vi "FFT_test.vi"() -> ()   [LabVIEW 2009]
uses:
  <vilib>/imath/engines/lvmath2/RunTimeEngine/ErrorHandling/NIMS_Finalize Error.vi
  <vilib>/imath/engines/lvmath2/RunTimeEngine/Parser/MC_Version.vi
  <vilib>/imath/engines/lvmath2/RunTimeEngine/NodeEndStatement/NIMS_NodeEndStatement_Output.vi
  <instcachedir>/0/NIMS_NodeEndStatement_Output_53EC0D466D134D7ABD903AC30B43404B.lvgen/NIMS_NodeEndStatement_Output_53EC0D466D134D7ABD903AC30B43404B_001.vi
  <vilib>/imath/engines/lvmath2/RunTimeEngine/RangeToken/NIMS_Range.vi
  <instcachedir>/0/NIMS_Range_08574DECC23E450FAF0AC0BC39E6BEA7.lvgen/NIMS_Range_08574DECC23E450FAF0AC0BC39E6BEA7_000.vi
  <vilib>/imath/engines/lvmath/Functions/Error Handling/MergeErrorsWrapper.vi
  <vilib>/imathl/engines/lvmath/Functions/Error Handling/Create Error.vi
  <vilib>/imath/engines/lvmath/Functions/Error Handling/MC_Error Cluster From Error Code.vi
  <vilib>/imath/engines/lvmath2/RunTimeEngine/BuiltInFunctions/randnormal/NIMS_randnormal(1,I32).vi
  <vilib>/imath/engines/lvmath2/RunTimeEngine/ArithmeticOperatorToken/NIMS_ArithmeticOperator_power(S).vi
  <instcachedir>/0/NIMS_ArithmeticOperator_power(S)_4AA2794EBDEE41D3AEDF40937D3906E7.lvgen/NIMS_ArithmeticOperator_power(S)_4AA2794EBDEE41D3AEDF40937D3906E7_001.vi
  <vilib>/imath/engines/lvmath2/RunTimeEngine/BuiltInFunctions/fft/NIMS_fft(GV).vi
  <instcachedir>/0/NIMS_fft(GV)_4C6467FC22F84E4BA42517A07EF978B0.lvgen/NIMS_fft(GV)_4C6467FC22F84E4BA42517A07EF978B0_001.vi
  <vilib>/imath/engines/lvmath2/RunTimeEngine/BuiltInFunctions/abs/NIMS_abs(signed).vi
  <instcachedir>/0/NIMS_abs(signed)_C4FCB8E6058B49B797C7C8D53CA5F6EC.lvgen/NIMS_abs(signed)_C4FCB8E6058B49B797C7C8D53CA5F6EC_000.vi
panel:
  out "FFT of 1023 Pt Sequence":cluster{dbl[], dbl[]}(graph)
  out "Time Domain Sequence":cluster{dbl[], dbl[]}(graph)
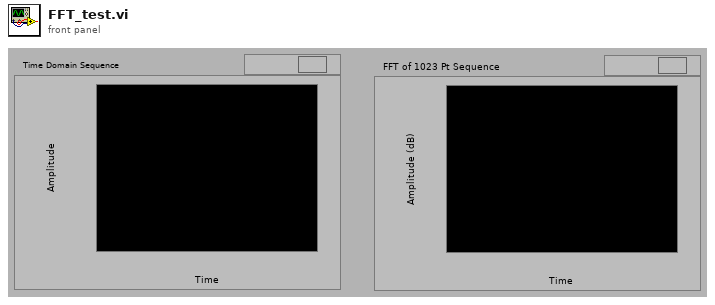
[diagram p1: front panel]
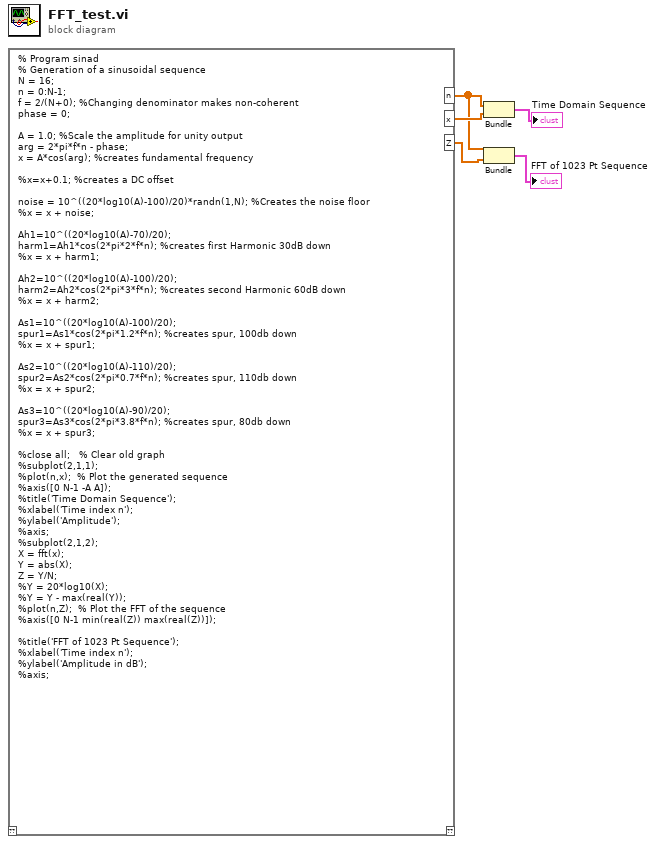
[diagram p0: block diagram]
diagram:
  n1 = mathscript code="% Program sinad\n% Generation of a sinusoidal sequence\nN = 16;\nn = 0:N-1;\t\nf = 2/(N+0); %Changing denominator makes non-coherent\nphase = 0;\t\t\t\n\nA = 1.0; %Scale the amplitude for unity output\narg = 2*pi*f*n - phase; \nx = A*cos(arg); %creates fundamental frequency\n\n%x=x+0.1; %creates a DC offset\n\nnoise = 10^((20*log10(A)-100)/20)*randn(1,N); %Creates the noise floor\n%x = x + noise;\n\nAh1=10^((20*log10(A)-70)/20);\nharm1=Ah1*cos(2*pi*2*f*n); %creates first Harmonic 30dB down\n%x = x + harm1;\n\nAh2=10^((20*log10(A)-100)/20);\nharm2=Ah2*cos(2*pi*3*f*n); %creates second Harmonic 60dB down\n%x = x + harm2;\n\nAs1=10^((20*log10(A)-100)/20);\nspur1=As1*cos(2*pi*1.2*f*n); %creates spur, 100db down\n%x = x + spur1;\n\nAs2=10^((20*log10(A)-110)/20);\nspur2=As2*cos(2*pi*0.7*f*n); %creates spur, 110db down\n%x = x + spur2;\n\nAs3=10^((20*log10(A)-90)/20);\nspur3=As3*cos(2*pi*3.8*f*n); %creates spur, 80db down\n%x = x + spur3;\n\n%close all;\t\t\t% Clear old graph\n%subplot(2,1,1);\n%plot(n,x);\t\t% Plot the generated sequence\n%axis([0 N-1 -A A]);\n%title('Time Domain Sequence');\n%xlabel('Time index n');\n%ylabel('Amplitude');\n%axis;\n%subplot(2,1,2);\nX = fft(x);\nY = abs(X);\nZ = Y/N;\n%Y = 20*log10(X);\n%Y = Y - max(real(Y));\n%plot(n,Z);\t\t% Plot the FFT of the sequence\n%axis([0 N-1 min(real(Z)) max(real(Z))]);\n \n%title('FFT of 1023 Pt Sequence');\n%xlabel('Time index n');\n%ylabel('Amplitude in dB');\n%axis;"() -> ("n"=w4:dbl[], "x"=w5:dbl[], "Z"=w3:dbl[])  [unwired: 1 in, 1 out]
  n2 = Bundle(w4, w5) -> (→"Time Domain Sequence":cluster{dbl[], dbl[]})  [unwired: 1 in]
  n3 = Bundle(w4, w3) -> (→"FFT of 1023 Pt Sequence":cluster{dbl[], dbl[]})  [unwired: 1 in]
